vi "__StripDataFromVAttributes.vi"(8 "error in (no error)":errorcluster, 11 "Map":variant) -> (0 "error out":errorcluster, 3 "duplicate variant":variant)   [LabVIEW 2019, in "lv-apt-json-file.lvlib"]
uses:
  lv-apt-json-file.lvlib
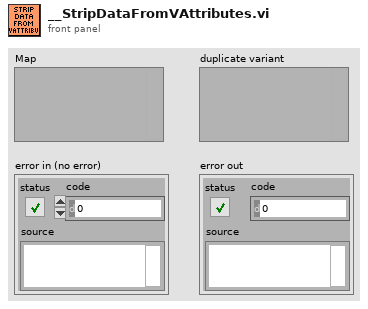
[diagram p1: front panel]
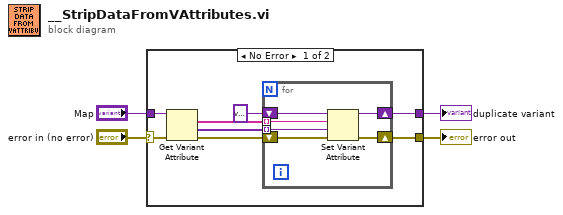
[diagram p0: block diagram]
diagram:
  n1 = case shown="No Error" "error in (no error)" {
    selector: "error in (no error)" -> [w12 w19]
    tunnel: [w10 w19] -> w3
    tunnel: [w9 _] -> w2
    tunnel: "Map" -> [w5 _]
    frame No Error {
      n2 = Get Variant Attribute(Variant=w5, error in=w12) -> (names=w7:string[], values=w8:variant[], error out=w11:errorcluster)  [unwired: 2 in, 1 out]
      n3 = for {
        shift-right: [w17] -> w9
        shift-left: variant ("duplicate variant") -> [w18]
        tunnel: w7 -> [w16] mode=indexing
        tunnel: w8 -> [w15] mode=indexing
        shift-right: [w14] -> w10
        shift-left: w11 -> [w13]
        n4 = Set Variant Attribute(Variant=w18, name=w16, value=w15, error in=w13) -> (Variant out=w17:variant, error out=w14:errorcluster)  [unwired: 1 out]
      }
    }
    frame Error {
    }
  }
  "error out" <- w3
  "duplicate variant" <- w2
